vi "Get Notification Name.vi"(11 "notification in":cluster{"value":variant, "name":string}) -> (2 "name":string, 3 "notification out":cluster{"value":variant, "name":string})   [LabVIEW 2014, in "Observable Actor.lvlib" / "Observable Actor.lvclass"]
uses:
  Observable Actor.lvclass
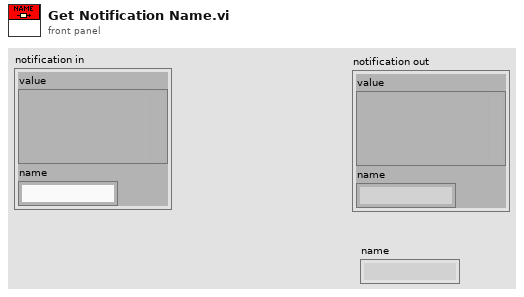
[diagram p1: front panel]
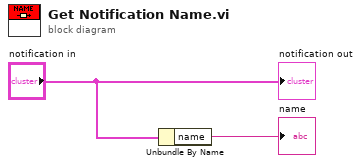
[diagram p0: block diagram]
diagram:
  n1 = Unbundle By Name("notification in") -> ("name"=→"name":string)
  "notification out" <- "notification in"
